vi "Do.vi"(8 "error in (no error)":errorcluster, 10 "Input":variant, 11 "Sample Temp PWM Control in":refnum<class "Sample Temp PWM Control.lvclass">) -> (0 "error out":errorcluster, 2 "Output":variant, 3 "Sample Temp PWM Control out":refnum<class "Sample Temp PWM Control.lvclass">)   [LabVIEW 2023, in "Sample Temp PWM Control.lvclass"]
uses:
  Sample Temp PWM Control.lvclass
  Sample Temp PWM Control.lvclass/Sample Temp PWM Control.ctl
  Task/Task Base/Task Base.lvclass
  Measure and Stimulus Subsystems/Measure and Stimulus Subsystems.lvclass
  <vilib>/addons/control/pid/NI_PID_pid.lvlib
  <vilib>/addons/control/pid/pid.llb/PID (DBL).vi
  D:/git/HAL/HAL GOOP4/Task/Task Base/Task Base.lvclass
  D:/git/HAL/HAL GOOP4/Tests/RT Tests/Sample Tasks/Sample Temp PWM Control/Sample Temp PWM Control.lvclass
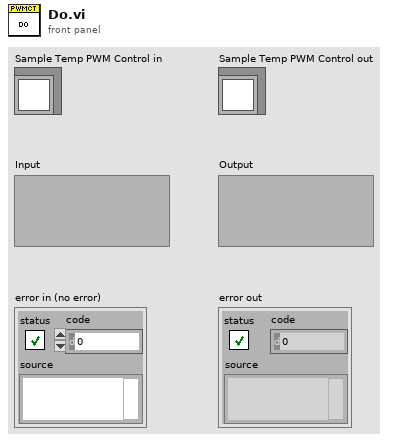
[diagram p1: front panel]
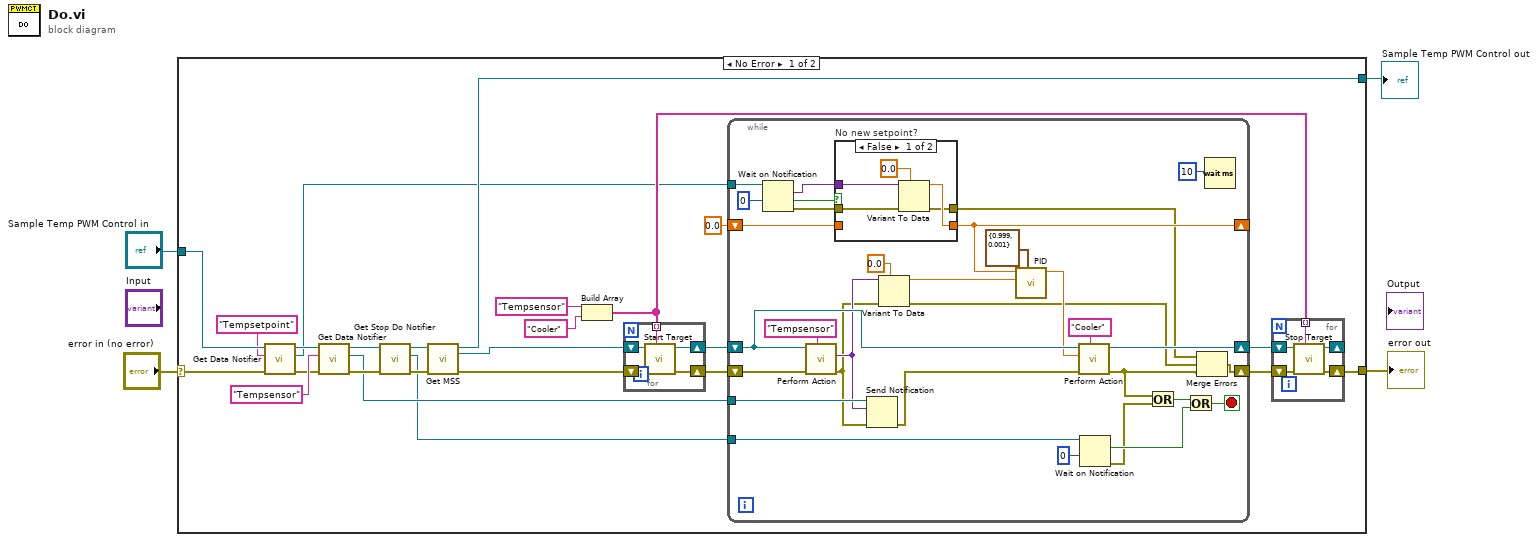
[diagram p0: block diagram]
diagram:
  n1 = case shown="No Error" "error in (no error)" {
    selector: "error in (no error)" -> [w26 w79]
    tunnel: [w22 w79] -> w1
    tunnel: [w14 w78] -> w2
    tunnel: "Sample Temp PWM Control in" -> [w9 w78]
    frame No Error {
      n2 = call "Get Data Notifier.vi"("error in (no error)"=w26, "Target Name"="Tempsetpoint", "Task Base in"=w9) -> ("error out"=w10:errorcluster, "Data Notifier"=w6:refnum<notifier>, "Task Base out"=w8:refnum<class "Sample Temp PWM Control.lvclass">)  [unwired: 6 in]
      n3 = call "Get Data Notifier.vi"("error in (no error)"=w10, "Target Name"="Tempsensor" ("Target Identifier"), "Task Base in"=w8) -> ("error out"=w16:errorcluster, "Data Notifier"=w15:refnum<notifier>, "Task Base out"=w13:refnum<class "Sample Temp PWM Control.lvclass">)  [unwired: 6 in]
      n4 = call "Get Stop Do Notifier.vi"("error in (no error)"=w16, "Task Base in"=w13) -> ("error out"=w21:errorcluster, "Stop Do"=w11:refnum<notifier>, "Task Base out"=w20:refnum<class "Sample Temp PWM Control.lvclass">)  [unwired: 7 in]
      n5 = call "Get MSS.vi"("error in (no error)"=w21, "Task Base in"=w20) -> ("error out"=w25:errorcluster, "MSS"=w24:refnum<class "Measure and Stimulus Subsystems.lvclass">, "Task Base out"=w14:refnum<class "Sample Temp PWM Control.lvclass">)  [unwired: 7 in]
      n6 = Build Array("Tempsensor" ("Target Identifier"), "Cooler" ("Target Identifier")) -> (w17:string[])
      n7 = for {
        shift-right: [w34] -> w29
        shift-left: w25 -> [w32]
        shift-right: [w33] -> w28
        shift-left: w24 -> [w31]
        tunnel: w17 -> [w30] mode=indexing
        n8 = call "Start Target.vi"("Target Ident"=w30, "Error In"=w32, "reference in"=w31) -> ("Error Out"=w34:errorcluster, "reference out"=w33:refnum<class "Measure and Stimulus Subsystems.lvclass">)  [unwired: 7 in]
      }
      n9 = while {
        shift-right: [w57] -> w27
        shift-left: w29 -> [w61]
        shift-right: [w63] -> w23
        shift-left: w28 -> [w60]
        tunnel: w15 -> [w51]
        tunnel: w11 -> [w48]
        tunnel: w6 -> [w45]
        shift-right: [w41] -> _
        shift-left: 0.0 -> [w38]
        stop <- w56 stop-if-true
        n10 = Wait on Notification(notifier=w45, timeout in ms (-1)=0) -> (notification=w43:variant, timed out?=w39:bool, error out=w44:errorcluster)  [unwired: 2 in, 1 out]
        n11 = call "Perform Action.vi"("Target Ident"="Tempsensor" ("Target Identifier"), "Error In"=w61, "reference in"=w60) -> ("Error Out"=w46:errorcluster, "Output"=w47:variant)  [unwired: 6 in, 1 out]
        n12 = case "No new setpoint?" shown="False" w39 {
          tunnel: w44 -> [w70 w72]
          tunnel: w43 -> [w69 _]
          tunnel: [w67 w71] -> w41
          tunnel: w38 -> [_ w71]
          tunnel: [w66 w72] -> w35
          frame False {
            n13 = Variant To Data(error in=w70, type=0.0, Variant=w69) -> (data=w67:dbl, error out=w66:errorcluster)
          }
          frame True {
          }
        }
        n14 = Send Notification(notification=w47, notifier=w51, error in (no error)=w46) -> (error out=w50:errorcluster)  [unwired: 1 out]
        n15 = Variant To Data(error in=w46, type=0.0, Variant=w47) -> (data=w59:dbl, error out=w36:errorcluster)
        n16 = call-poly <vilib>:"PID.vi"("output range"=cluster{"output high":dbl, "output low":dbl} {"output high"=0.999, "output low"=0.001}, "process variable"=w59, "setpoint"=w41) -> ("output"=w58:dbl)  [unwired: 7 in, 1 out]
        n17 = call "Perform Action.vi"("Target Ident"="Cooler", "Error In"=w50, "Input"=w58, "reference in"=w60) -> ("Error Out"=w37:errorcluster, "reference out"=w63:refnum<class "Measure and Stimulus Subsystems.lvclass">)  [unwired: 5 in, 1 out]
        n18 = Wait on Notification(notifier=w48, timeout in ms (-1)=0) -> (notification=w54:bool, error out=w53:errorcluster)  [unwired: 2 in, 2 out]
        n19 = Or(x=w37, y=w53) -> (x .or. y?=w52:bool)
        n20 = Or(x=w52, y=w54) -> (x .or. y?=w56:bool)
        n21 = Merge Errors(w35, w36, w37) -> (w57:errorcluster)
        n22 = Wait (ms)(milliseconds to wait=u32 10) -> ()  [unwired: 1 out]
      }
      n23 = for {
        shift-right: [w75] -> w22
        shift-left: w27 -> [w77]
        tunnel: w17 -> [w74] mode=indexing
        shift-right: [w73] -> _
        shift-left: w23 -> [w76]
        n24 = call "Stop Target.vi"("Target Ident"=w74, "Error In"=w77, "reference in"=w76) -> ("Error Out"=w75:errorcluster, "reference out"=w73:refnum<class "Measure and Stimulus Subsystems.lvclass">)  [unwired: 7 in]
      }
    }
    frame Error {
    }
  }
  "error out" <- w1
  "Sample Temp PWM Control out" <- w2
